vi "report_module.vi"(0 "limits":T3, 1 "mode":T1, 5 "data":T2, 11 "error in (no error)":errorcluster) -> (4 "Torque":bool, 6 "Passed":bool, 8 "Rpm":bool, 10 "Efficiency":bool, 14 "step status":bool, 15 "error out":errorcluster)   [LabVIEW 2019]
uses:
  limits_limitList.ctl
  limits_specs.ctl
  core/core_autoMonitorDataCluster.ctl
  report_mode.ctl
  Write Mode.ctl
  Read Mode.ctl
  part number.vi
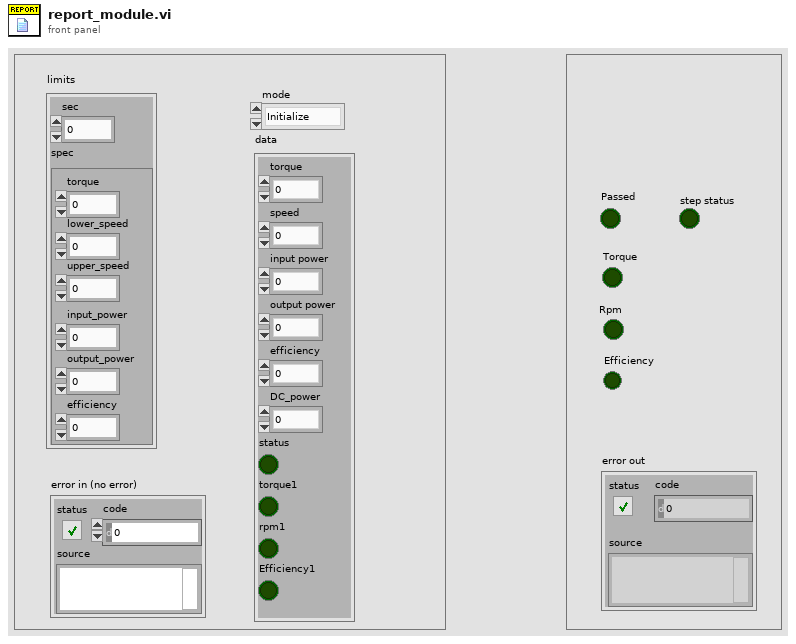
[diagram p1: front panel]
types:
  T1 = typedef "report_mode.ctl" = enum16{"Initialize", "Save", "Close"}
  T2 = typedef "core_autoMonitorDataCluster.ctl" = cluster{"torque":dbl, "speed":dbl, "input power":dbl, "output power":dbl, "efficiency":dbl, "DC_power":dbl, "status":bool, "torque1":bool, "rpm1":bool, "Efficiency1":bool}
  T3 = typedef "limits_limitList.ctl" = cluster{"sec":i32, "spec":T4}
  T4 = typedef "limits_specs.ctl" = cluster{"torque":dbl, "lower_speed":dbl, "upper_speed":dbl, "input_power":dbl, "output_power":dbl, "efficiency":dbl}
  T5 = typedef "Read Mode.ctl" = enum16{"PLC_to_PC", "Partnumber_to_PC", "Initialize", "Close"}
  T6 = typedef "Write Mode.ctl" = enum16{"GetRef", "Initialize", "Close"}
  T7 = enum16{"open", "replace", "create", "open or create", "replace or create", "replace or create with confirmation"}
  T8 = typedef "save.ctl" = string
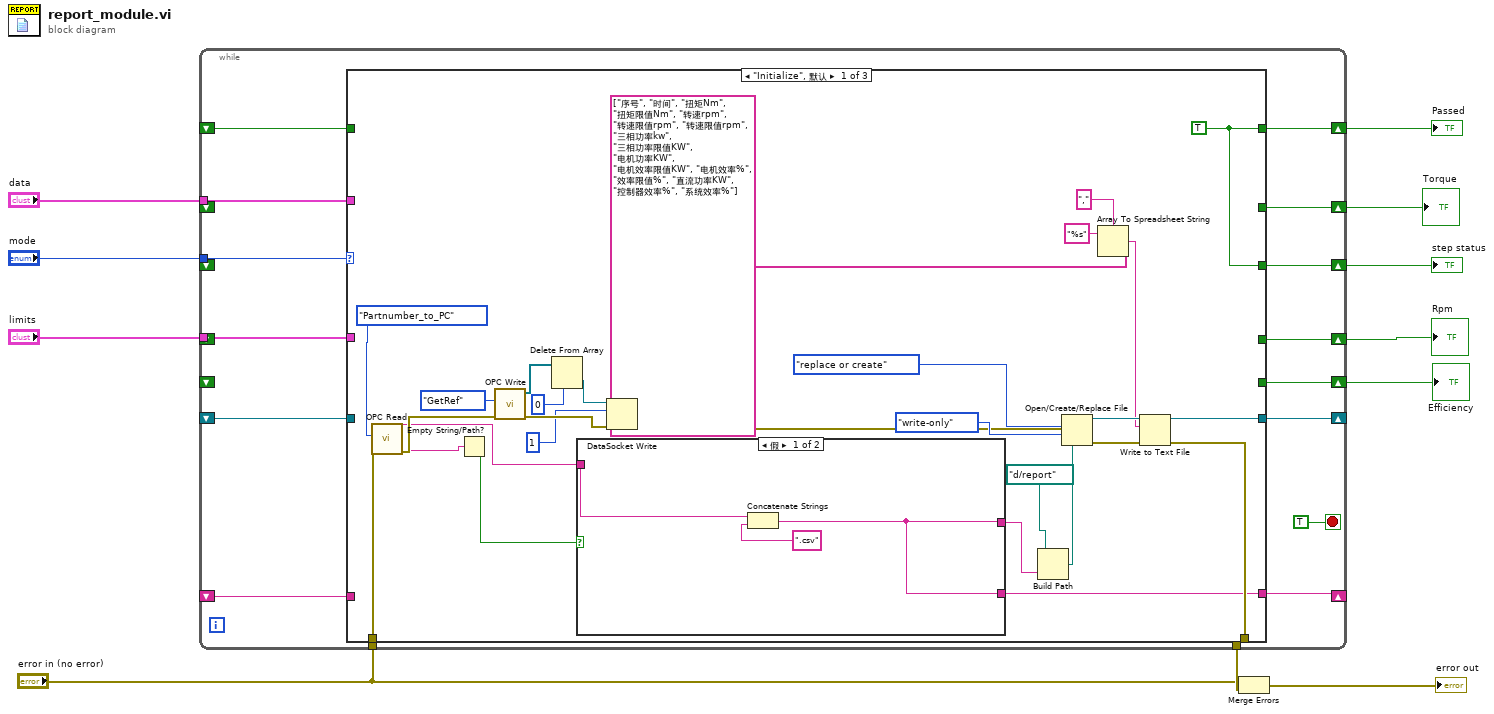
[diagram p0: block diagram]
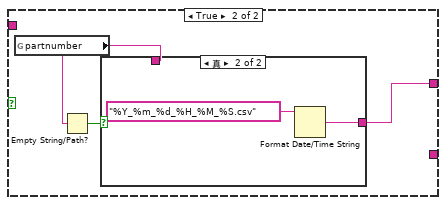
[diagram p2: hidden frame]
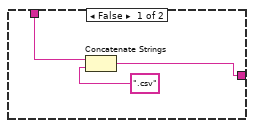
[diagram p3: hidden frame]
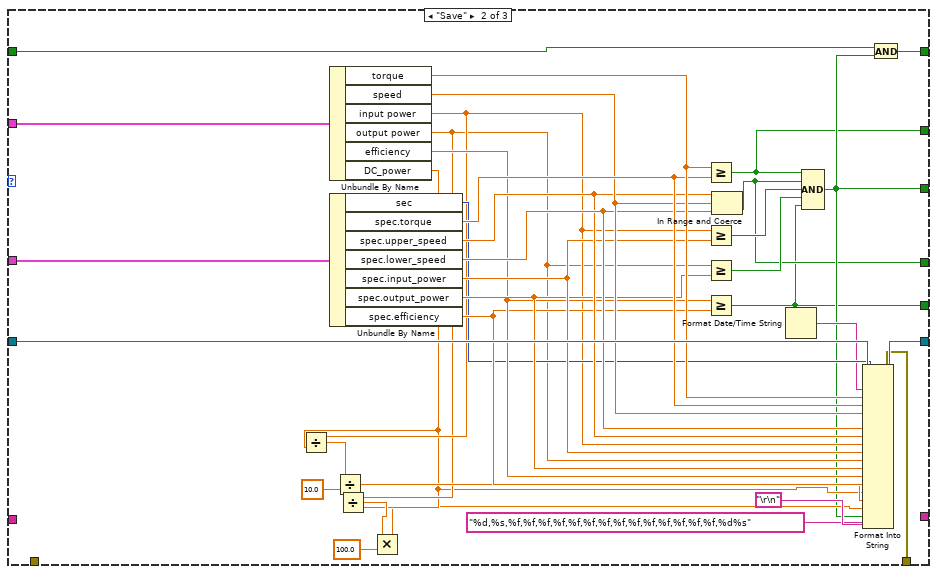
[diagram p4: hidden frame]
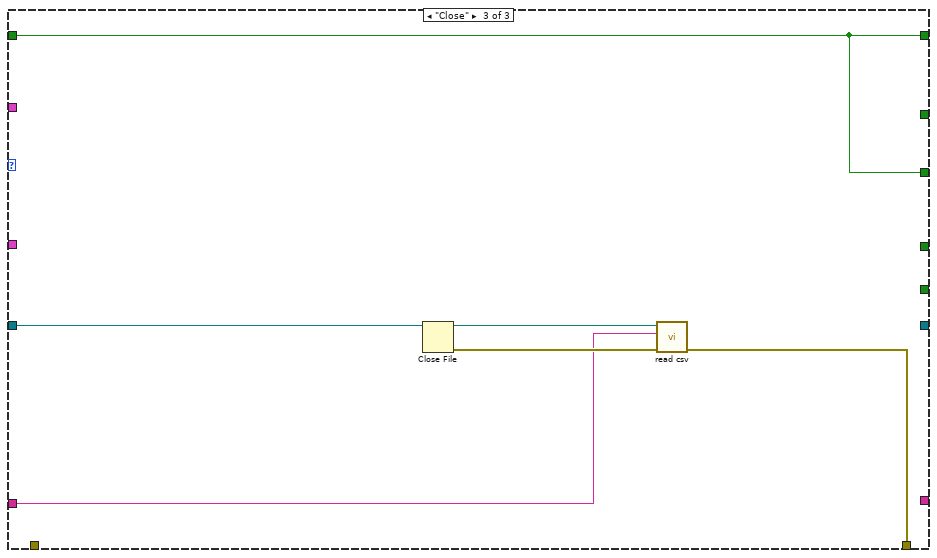
[diagram p5: hidden frame]
diagram:
  n1 = while {
    tunnel: "data" -> [w26]
    tunnel: "limits" -> [w25]
    tunnel: "mode" -> [w24]
    shift-right: [w27] -> w11
    shift-left: _ -> [w22]
    shift-right: [w21] -> _
    shift-left: _ -> [w20]
    tunnel: [w19] -> w6
    shift-right: [w17] -> _
    shift-left: _ -> [w16]
    tunnel: "error in (no error)" -> [w15]
    shift-right: [w18] -> w5
    shift-left: _ -> [_]
    shift-right: [w13] -> w2
    shift-left: _ -> [_]
    shift-right: [w12] -> w1
    shift-left: _ -> [_]
    shift-right: [w14] -> w3
    shift-left: _ -> [_]
    stop <- TRUE stop-if-true
    n2 = case shown="\"Initialize\", 默认" w24 {
      tunnel: [w45 w95 w105] -> w27
      tunnel: w26 -> [_ w98 _]
      tunnel: w25 -> [_ w97 _]
      tunnel: w22 -> [_ w96 w105]
      tunnel: [w52 w93 _] -> w21
      tunnel: w20 -> [_ w94 w106]
      tunnel: [w50 w83 w102] -> w19
      tunnel: [w45 w69 w105] -> w18
      tunnel: [w39 _ _] -> w17
      tunnel: w16 -> [_ _ w101]
      tunnel: w15 -> [w28 _ _]
      tunnel: [_ w68 _] -> w14
      tunnel: [_ w67 _] -> w13
      tunnel: [_ w66 _] -> w12
      frame "Initialize", Default {
        w45 = TRUE
        n3 = call "OPC Read.vi"("error in (no error)"=w28, "Mode"=Read_Mode."Partnumber_to_PC") -> ("error out"=w31:errorcluster, "date"=w30:string)  [unwired: 5 in, 3 out]
        n4 = Empty String/Path?(string/path=w30) -> (empty?=w42:bool)
        n5 = call "OPC Write.vi"("error in (no error)"=w31, "Mode"=Write_Mode."GetRef") -> ("error out"=w34:errorcluster, "all ref"=w36:refnum<k13>[])  [unwired: 7 in, 1 out]
        n6 = Delete From Array(array=w36, index=0 ("索引")) -> (deleted portion=w35:refnum<k13>)  [unwired: 1 in, 1 out]
        n7 = case shown="假" w42 {
          tunnel: [w55 w60] -> w40
          tunnel: w30 -> [w56 _]
          tunnel: [w55 _] -> w39
          frame False {
            n8 = Concatenate Strings(w56, ".csv" ("time format string (%c)")) -> (w55:string)
          }
          frame True {
            n9 = global read "part number.vi" "partnumber"() -> (w58:T8)
            n10 = Empty String/Path?(string/path=w58) -> (empty?=w59:bool)
            n11 = case shown="真" w59 {
              tunnel: [w62 w65] -> w60
              tunnel: w58 -> [w61 _]
              frame False {
                n12 = Concatenate Strings(w61, ".csv" ("time format string (%c)")) -> (w62:string)
              }
              frame True {
                n13 = Format Date/Time String(time format string (%c)="%Y_%m_%d_%H_%M_%S.csv") -> (date/time string=w65:string)  [unwired: 2 in]
              }
            }
          }
        }
        n14 = DataSocket Write(8:w34, 10:1 ("索引"), 11:w35) -> (0:w33:errorcluster)  [unwired: 1 in, 2 out]
        n15 = Build Path(base path=path "d:/report", name or relative path=w40) -> (appended path=w41:path)
        n16 = Open/Create/Replace File(file path (use dialog)=w41, error in=w33, operation (0:open)=T7."replace or create", access (0:read/write)=enum16{"read/write", "read-only", "write-only"}."write-only") -> (refnum out=w54:refnum<file>, error out=w51:errorcluster)  [unwired: 2 in, 1 out]
        n17 = Array To Spreadsheet String(delimiter (Tab)=",", array=string[] ["序号", "时间", "扭矩Nm", "扭矩限值Nm", "转速rpm", "转速限值rpm", "转速限值rpm", "三相功率kw", "三相功率限值KW", "电机功率KW", "电机效率限值KW", "电机效率%", "效率限值%", "直流功率KW", "控制器效率%", "系统效率%"], 3:"%s" ("format string")) -> (spreadsheet string=w48:string)
        n18 = Write to Text File(file (use dialog)=w54, text=w48, error in=w51) -> (refnum out=w52:refnum<file>, error out=w50:errorcluster)  [unwired: 1 in, 1 out]
      }
      frame "Save" {
        n19 = Unbundle By Name(w98) -> ("torque"=w92:dbl, "speed"=w90:dbl, "input power"=w76:dbl, "output power"=w72:dbl, "efficiency"=w85:dbl, "DC_power"=w71:dbl)
        n20 = Divide(x=w76, y=w71) -> (x/y=w78:dbl)
        n21 = Unbundle By Name(w97) -> ("sec"=w82:i32, "spec.torque"=w91:dbl, "spec.upper_speed"=w88:dbl, "spec.lower_speed"=w89:dbl, "spec.input_power"=w87:dbl, "spec.output_power"=w86:dbl, "spec.efficiency"=w84:dbl)
        n22 = Divide(x=w78, y=10.0) -> (x/y=w75:dbl)
        n23 = Divide(x=w72, y=w71) -> (x/y=w73:dbl)
        n24 = Multiply(x=w73, y=100.0) -> (x*y=w70:dbl)
        n25 = Greater Or Equal?(x=w92, y=w91) -> (x >= y?=w68:bool)
        n26 = Greater Or Equal?(x=w76, y=w87) -> (x >= y?=w100:bool)
        n27 = Greater Or Equal?(x=w72, y=w86) -> (x >= y?=w99:bool)
        n28 = Greater Or Equal?(x=w85, y=w84) -> (x >= y?=w66:bool)
        n29 = In Range and Coerce(upper limit=w88, x=w90, lower limit=w89) -> (In Range?=w67:bool)  [unwired: 1 out]
        n30 = Format Date/Time String() -> (date/time string=w79:string)  [unwired: 3 in]
        n31 = Compound Arithmetic op=AND(w68, w67, w100, w99, w66) -> (w69:bool)
        n32 = Format Into String(format string="%d,%s,%f,%f,%f,%f,%f,%f,%f,%f,%f,%f,%f,%f,%f,%f,%d%s", initial string=w94, w82, w79, w92, w91, w90, w89, w88, w76, w87, w72, w86, w85, w84, w71, w75, w70, w69, "\r\n") -> (resulting string=w93:refnum<file>, error out=w83:errorcluster)  [unwired: 1 in]
        n33 = And(x=w96, y=w69) -> (x .and. y?=w95:bool)
      }
      frame "Close" {
        n34 = Close File(refnum=w106) -> (path=w103:path, error out=w104:errorcluster)  [unwired: 1 in]
        n35 = call "read csv.vi"("error in (no error)"=w104, "String"=w101, "Path"=w103) -> ("error out"=w102:errorcluster)  [unwired: 8 in]
      }
    }
  }
  "Passed" <- w11
  "step status" <- w5
  "Rpm" <- w2
  "Torque" <- w3
  "Efficiency" <- w1
  n36 = Merge Errors("error in (no error)", w6) -> (→"error out":errorcluster)
